vi "Get Application Version.vi"() -> (1 "run time system":bool, 2 "last mod":timestamp, 3 "version string":string, 4 "app. version number":string)   [LabVIEW 2013, in "varilib.lvlib"]
doc: "Returns application version number and last modification date for compiled exe file. In the case of developement or other, returns describing text."
uses:
  varilib.lvlib
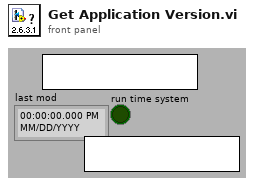
[diagram p1: front panel]
types:
  T1 = enum32{"invalid app kind", "Development System", "Run Time System", "Student Edition", "Embedded LabVIEW", "Evaluation", "Custom"}
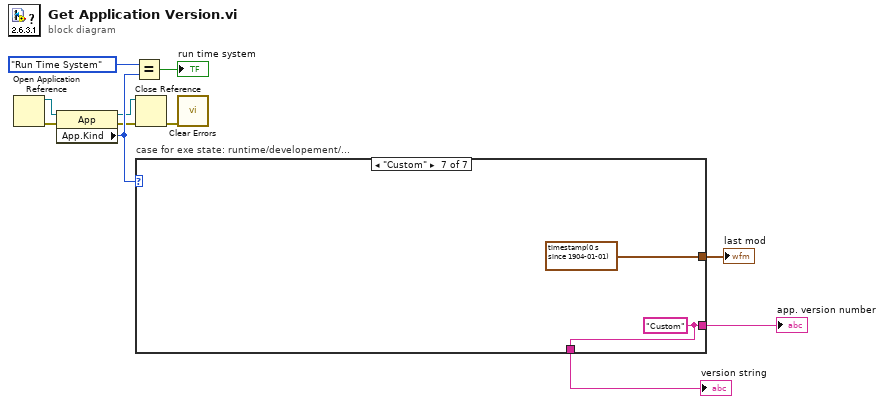
[diagram p0: block diagram]
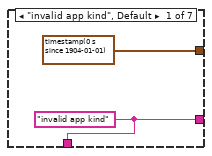
[diagram p2: hidden frame]
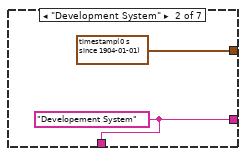
[diagram p3: hidden frame]
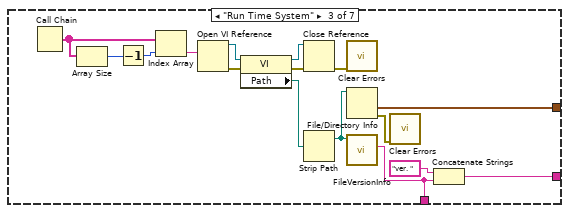
[diagram p4: hidden frame]
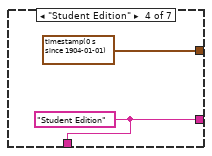
[diagram p5: hidden frame]
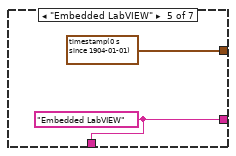
[diagram p6: hidden frame]
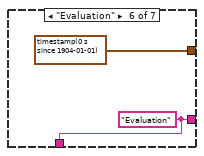
[diagram p7: hidden frame]
diagram:
  n1 = Open Application Reference() -> (0:w7:errorcluster, 3:w11:refnum<vi>)  [unwired: 4 in]
  n2 = property class="App"(reference=w11, error in=w7) -> (reference out=w5:refnum<vi>, error out=w6:errorcluster, "App.Kind"=w9:T1)
  n3 = Equal?(x=T1."Run Time System" ("Application:Kind"), y=w9) -> (x = y?=→"run time system":bool)
  n4 = Close Reference(reference=w5, error in (no error)=w6) -> (error out=w3:errorcluster)
  n5 = case "case for exe state: runtime/developement/..." shown="\"Custom\"" w9 {
    tunnel: [w12 w14 w30 w32 w34 w36 w38] -> w2
    tunnel: [timestamp(0 s since 1904-01-01) ("last mod") timestamp(0 s since 1904-01-01) ("last mod") w19 timestamp(0 s since 1904-01-01) ("last mod") timestamp(0 s since 1904-01-01) ("last mod") timestamp(0 s since 1904-01-01) ("last mod") timestamp(0 s since 1904-01-01) ("last mod")] -> w4
    tunnel: [w12 w14 w16 w32 w34 w36 w38] -> w1
    frame "invalid app kind", Default {
      w12 = "invalid app kind"
    }
    frame "Development System" {
      w14 = "Developement System"
    }
    frame "Run Time System" {
      n6 = Call Chain() -> (call chain=w26:string[])
      n7 = Array Size(array=w26) -> (size(s)=w27:i32)
      n8 = Decrement(x=w27) -> (x-1=w25:i32)
      n9 = Index Array(array=w26, index=w25) -> (element=w24:string)
      n10 = Open VI Reference(vi path=w24) -> (vi reference=w28:refnum<vi>, error out=w29:errorcluster)  [unwired: 5 in]
      n11 = property class="VI"(reference=w28, error in=w29) -> (reference out=w22:refnum<vi>, error out=w23:errorcluster, "Path"=w21:path)
      n12 = Close Reference(reference=w22, error in (no error)=w23) -> (error out=w17:errorcluster)
      n13 = Strip Path(path=w21) -> (stripped path=w20:path)  [unwired: 1 out]
      n14 = call <vilib>:"Clear Errors.vi"("error in (no error)"=w17) -> ()  [unwired: 6 in, 1 out]
      n15 = File/Directory Info(path=w20) -> (last mod=w19:timestamp, error out=w18:errorcluster)  [unwired: 1 in, 5 out]
      n16 = call <vilib>:"FileVersionInfo.vi"("Application Path in"=w20) -> ("File Version Info"=w16:string)  [unwired: 7 in, 3 out]
      n17 = call <vilib>:"Clear Errors.vi"("error in (no error)"=w18) -> ()  [unwired: 6 in, 1 out]
      n18 = Concatenate Strings("ver. " ("string"), w16) -> (w30:string)
    }
    frame "Student Edition" {
      w32 = "Student Edition"
    }
    frame "Embedded LabVIEW" {
      w34 = "Embedded LabVIEW"
    }
    frame "Evaluation" {
      w36 = "Evaluation"
    }
    frame "Custom" {
      w38 = "Custom"
    }
  }
  "app. version number" <- w2
  "last mod" <- w4
  "version string" <- w1
  n19 = call <vilib>:"Clear Errors.vi"("error in (no error)"=w3) -> ()  [unwired: 6 in, 1 out]
